vi "get coil current bool signs.vi"(9 "X current (mA)":dbl=70.0, 10 "Y current (mA)":dbl=-1980.0, 11 "Z current (mA)":dbl=-1155.0) -> (1 "x sign":bool=TRUE, 2 "y sign":bool, 3 "z sign":bool)   [LabVIEW 2018]
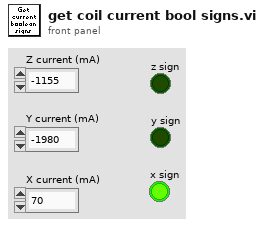
[diagram p1: front panel]
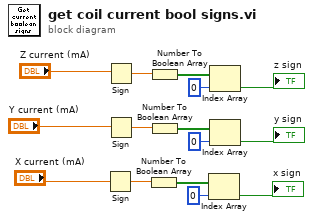
[diagram p0: block diagram]
diagram:
  n1 = Sign(1:"X current (mA)") -> (0:w6:dbl)
  n2 = Sign(1:"Z current (mA)") -> (0:w15:dbl)
  n3 = Sign(1:"Y current (mA)") -> (0:w7:dbl)
  n4 = Number To Boolean Array(number=w6) -> (Boolean array=w5:bool[])
  n5 = Number To Boolean Array(number=w15) -> (Boolean array=w14:bool[])
  n6 = Number To Boolean Array(number=w7) -> (Boolean array=w8:bool[])
  n7 = Index Array(array=w5, index=0) -> (element=→"x sign":bool)
  n8 = Index Array(array=w14, index=0) -> (element=→"z sign":bool)
  n9 = Index Array(array=w8, index=0) -> (element=→"y sign":bool)
